vi "Sound_Sub.vi"(0 "path":path) -> ()   [LabVIEW 2014]
uses:
  <vilib>/sound2/lvsound2.llb/Sampling Mode.ctl
  <vilib>/sound2/lvsound2.llb/Sound File Info (path).vi
  <vilib>/sound2/lvsound2.llb/Sound File Read Open.vi
  <vilib>/sound2/lvsound2.llb/Sound File Read (DBL).vi
  <vilib>/sound2/lvsound2.llb/Sound Output Write (DBL).vi
panel:
  in  "Stop":bool
  out "Current Iteration":i32
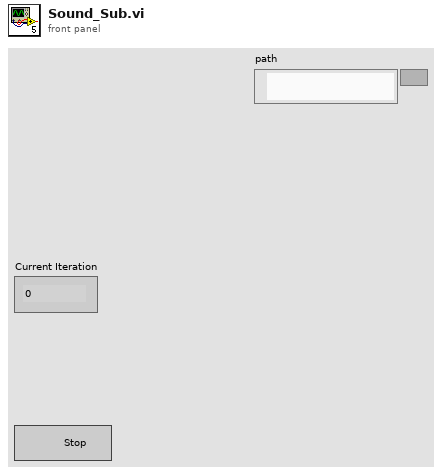
[diagram p1: front panel]
types:
  T1 = typedef "Sampling Mode.ctl" = i32
  T2 = typedef "Sound Data Format.ctl" = cluster{"sample rate (S/s)":dbl, "number of channels":i32, "bits per sample":i32}
  T3 = typedef "Sound File Refnum.ctl" = refnum<file>
  T4 = typedef "Sound Output Task ID.ctl" = u32
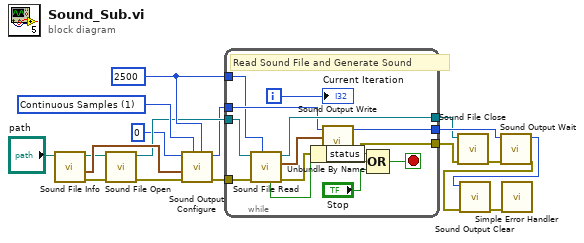
[diagram p0: block diagram]
diagram:
  w16 = 2500 ("Number of Samples/Iteration")
  w17 = T1 1 items=["Finite Samples", "Continuous Samples"] ("sample mode")
  n1 = call-poly <vilib>:"Sound File Info.vi"("path"="path") -> ("error out"=w8:errorcluster, "sound format"=w15:T2, "path out"=w14:path)  [unwired: 7 in, 1 out]
  n2 = call-poly <vilib>:"Sound File Open.vi"("error in (no error)"=w8, "path"=w14) -> ("error out"=w9:errorcluster, "sound file refnum"=w7:T3)  [unwired: 8 in]
  n3 = call <vilib>:"Sound Output Configure.vi"("number of samples/ch"=w16, "sample mode"=w17, "error in (no error)"=w9, "sound format"=w15, "device ID"=u32 0 ("Device ID")) -> ("error out"=w10:errorcluster, "task ID"=w3:T4)  [unwired: 5 in]
  n4 = while {
    tunnel: w16 -> [w22]
    tunnel: w7 -> [w30]
    tunnel: [w28] -> w5
    tunnel: w10 -> [w31]
    tunnel: [w21] -> w6
    tunnel: w3 -> [w27]
    tunnel: [w32] -> w11
    i -> [w29]
    stop <- w23 stop-if-true
    # "Read Sound File and Generate Sound"
    n5 = call-poly <vilib>:"Sound File Read.vi"("number of samples/ch (-1: all)"=w22, "error in (no error)"=w31, "sound file refnum"=w30) -> ("error out"=w26:errorcluster, "data"=w20:waveform(dbl)[], "sound file refnum out"=w28:T3, "end of file?"=w24:bool)  [unwired: 4 in, 1 out]
    n6 = call-poly <vilib>:"Sound Output Write.vi"("error in (no error)"=w26, "data"=w20, "task ID"=w27) -> ("error out"=w21:errorcluster, "task ID out"=w32:T4)  [unwired: 7 in]
    n7 = Unbundle By Name(w21) -> ("status"=w19:bool)
    n8 = Compound Arithmetic op=OR(w19, w24, "Stop") -> (w23:bool)
    "Current Iteration" <- w29
  }
  n9 = call <vilib>:"Sound File Close.vi"("error in (no error)"=w6, "sound file refnum"=w5) -> ("error out"=w12:errorcluster)  [unwired: 9 in]
  n10 = call <vilib>:"Sound Output Wait.vi"("error in (no error)"=w12, "task ID"=w11) -> ("error out"=w13:errorcluster, "task ID out"=w1:T4)  [unwired: 8 in]
  n11 = call <vilib>:"Sound Output Clear.vi"("error in (no error)"=w13, "task ID"=w1) -> ("error out"=w18:errorcluster)  [unwired: 9 in]
  n12 = call <vilib>:"Simple Error Handler.vi"("error in (no error)"=w18) -> ()  [unwired: 4 in, 5 out]
